vi "Cross-Bridge.vi"(7 "X-Y-Z移動":dbl[](array[numeric])=[1.0, 325.0, 0.0], 8 "Error In":errorcluster, 9 "動作":enum16{"補後退", "跳過"}(ring), 11 "校正選擇":enum16{"左前", "オ"}(ring)) -> (0 "Error Out":errorcluster)   [LabVIEW 2019]
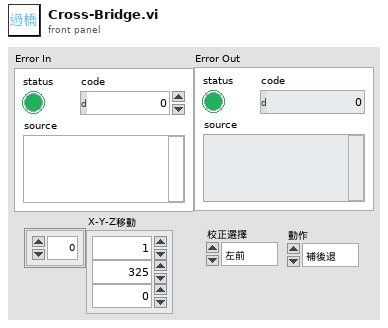
[diagram p1: front panel]
types:
  T1 = enum16{"前", "後", "オ", "右", "無", "0", "1", "2", "3", "4", "5", "6", "7"}
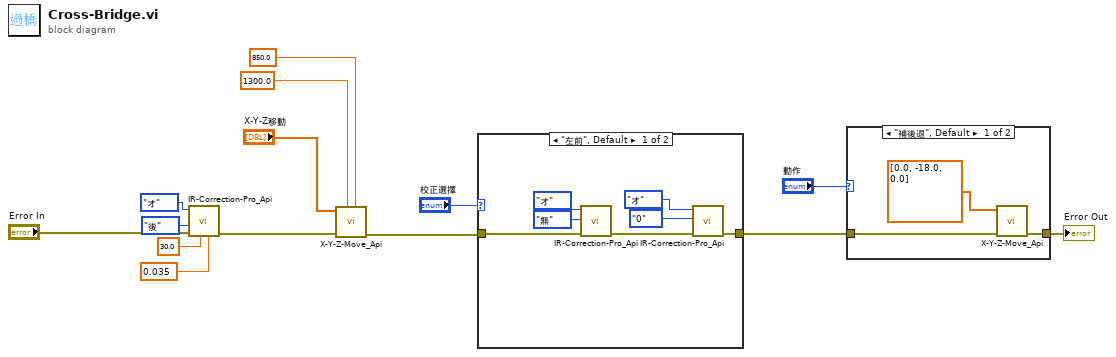
[diagram p0: block diagram]
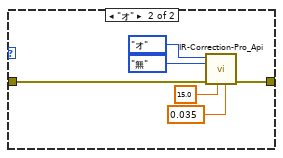
[diagram p2: hidden frame]
diagram:
  n1 = call "IR-Correction-Pro_Api.vi"("ExitRange"=0.035, "精準度"=30.0, "Error In"="Error In", "副邊校正"=T1."後", "主編校正"=enum16{"前", "後", "オ", "右", "無"}."オ") -> ("Error Out"=w8:errorcluster)  [unwired: 6 in]
  n2 = call "X-Y-Z-Move_Api.vi"("加速度"=850.0, "最高速"=1300.0, "Error In"=w8, "X-Y-Z移動"="X-Y-Z移動") -> ("Error Out"=w7:errorcluster)  [unwired: 6 in, 1 out]
  n3 = case shown="\"左前\", Default" "校正選擇" {
    tunnel: w7 -> [w17 w26]
    tunnel: [w21 w25] -> w13
    frame "左前", Default {
      n4 = call "IR-Correction-Pro_Api.vi"("Error In"=w17, "副邊校正"=T1."無", "主編校正"=enum16{"前", "後", "オ", "右", "無"}."オ") -> ("Error Out"=w18:errorcluster)  [unwired: 8 in]
      n5 = call "IR-Correction-Pro_Api.vi"("Error In"=w18, "副邊校正"=T1."0", "主編校正"=enum16{"前", "後", "オ", "右", "無"}."オ") -> ("Error Out"=w21:errorcluster)  [unwired: 8 in]
    }
    frame "オ" {
      n6 = call "IR-Correction-Pro_Api.vi"("ExitRange"=0.035, "精準度"=15.0, "Error In"=w26, "副邊校正"=T1."無", "主編校正"=enum16{"前", "後", "オ", "右", "無"}."オ") -> ("Error Out"=w25:errorcluster)  [unwired: 6 in]
    }
  }
  n7 = case shown="\"補後退\", Default" "動作" {
    tunnel: w13 -> [w30 w31]
    tunnel: [w29 w31] -> w12
    frame "補後退", Default {
      n8 = call "X-Y-Z-Move_Api.vi"("Error In"=w30, "X-Y-Z移動"=dbl[] [0.0, -18.0, 0.0]) -> ("Error Out"=w29:errorcluster)  [unwired: 8 in, 1 out]
    }
    frame "跳過" {
    }
  }
  "Error Out" <- w12
